vi "Write configuration.vi"(8 "error in":errorcluster, 10 "configuration":refnum<class "NISE_CEF_serializable configuration.lvclass">, 11 "TEST EDITOR in":refnum<class "TEST EDITOR.lvclass">) -> (0 "error out":errorcluster, 3 "TEST EDITOR out":refnum<class "TEST EDITOR.lvclass">)   [LabVIEW 2013, in "configuration tests.lvlib" / "TEST EDITOR.lvclass"]
uses:
  TEST EDITOR.lvclass
  <vilib>/NI/Configuration Framework/serializable configuration/NISE_CEF_serializable configuration.lvclass
  module/configuration/TEST CONFIGURATION.lvclass
  TEST EDITOR.lvclass/TEST EDITOR.ctl
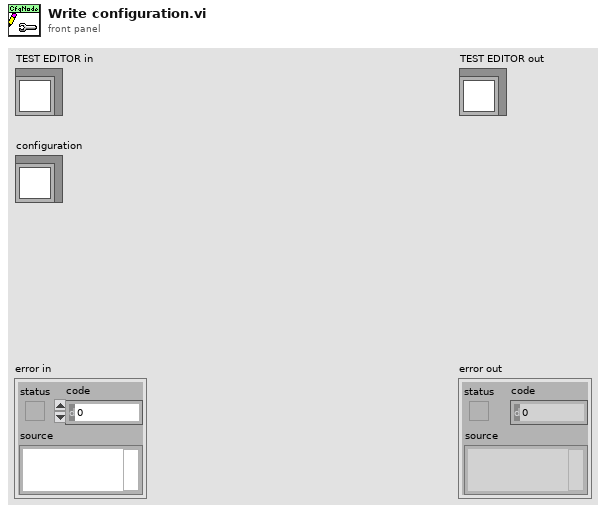
[diagram p1: front panel]
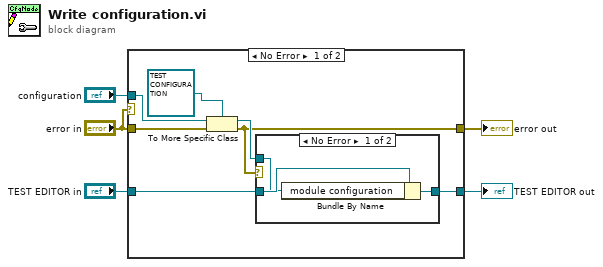
[diagram p0: block diagram]
diagram:
  n1 = case shown="No Error" "error in" {
    tunnel: "TEST EDITOR in" -> [w12 w18]
    tunnel: [w11 w18] -> w4
    tunnel: "configuration" -> [w8 _]
    tunnel: "error in" -> [w7 w17]
    tunnel: [w6 w17] -> w2
    frame No Error {
      n2 = To More Specific Class(target class=refnum<class "TEST CONFIGURATION.lvclass"> refnum ("module configuration"), reference=w8, error in=w7) -> (specific class reference=w9:refnum<class "TEST CONFIGURATION.lvclass">, error out=w6:errorcluster)
      n3 = case shown="No Error" w6 {
        tunnel: w12 -> [w15 w16]
        tunnel: [w14 w16] -> w11
        tunnel: w9 -> [w13 _]
        frame No Error {
          n4 = Bundle By Name(cluster=w15, "module configuration"=w13) -> (w14:refnum<class "TEST EDITOR.lvclass">)
        }
        frame Error {
        }
      }
    }
    frame Error {
    }
  }
  "error out" <- w2
  "TEST EDITOR out" <- w4
